vi "Class Method Property File Paths.vi"(8 "error in (no error)":errorcluster) -> (0 "error out":errorcluster, 1 "Method Ini":path, 2 "Property Ini":path, 3 "Class Ini":path, 4 "Files Found Cluster":T1)   [LabVIEW 2023]
doc: "Return paths to class/property/methods xml support files based on the current LV version"
uses:
  <userlib>/_OpenG.lib/file/file.llb/openg_file.lvlib
panel:
  out "file names":string[](array[string])
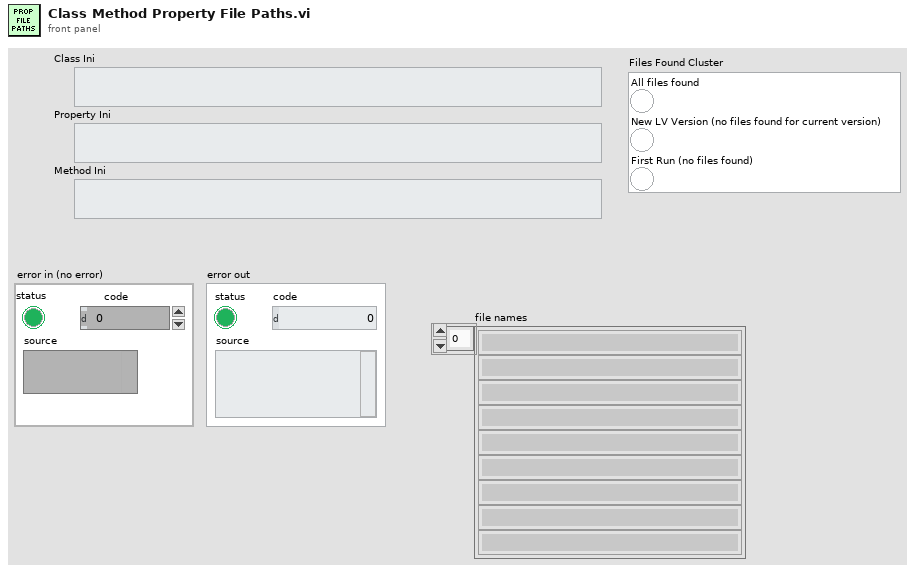
[diagram p1: front panel]
types:
  T1 = cluster{"All files found":bool, "New LV Version (no files found for current version)":bool, "First Run (no files found)":bool}
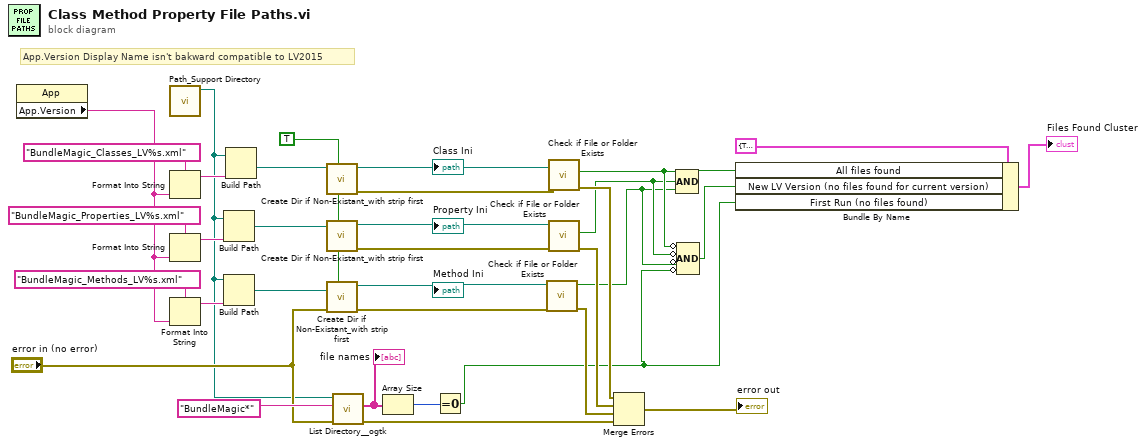
[diagram p0: block diagram]
diagram:
  w25 = TRUE ("Strip Path First [F]")
  # "App.Version Display Name isn't bakward compatible to LV2015"
  n1 = property class="App"() -> ("App.Version"=w35:string)  [unwired: 2 in, 2 out]
  n2 = call "Path_Support Directory.vi"() -> ("Support Directory"=w7:path)  [unwired: 11 in]
  n3 = Format Into String(format string="BundleMagic_Classes_LV%s.xml", w35) -> (resulting string=w30:string)  [unwired: 2 in, 1 out]
  n4 = Format Into String(format string="BundleMagic_Properties_LV%s.xml", w35) -> (resulting string=w31:string)  [unwired: 2 in, 1 out]
  n5 = Format Into String(format string="BundleMagic_Methods_LV%s.xml", w35) -> (resulting string=w34:string)  [unwired: 2 in, 1 out]
  n6 = Build Path(base path=w7, name or relative path=w31) -> (appended path=w27:path)
  n7 = Build Path(base path=w7, name or relative path=w34) -> (appended path=w26:path)
  n8 = Build Path(base path=w7, name or relative path=w30) -> (appended path=w28:path)
  n9 = call "Create Dir if Non-Existant_with strip first.vi"("Strip Path First [F]"=w25, "Directory Path"=w28) -> ("error out"=w21:errorcluster, "dup Directory Path"=w24:path)  [unwired: 7 in, 1 out]
  "Class Ini" <- w24
  n10 = call "Create Dir if Non-Existant_with strip first.vi"("Strip Path First [F]"=w25, "Directory Path"=w27) -> ("error out"=w20:errorcluster, "dup Directory Path"=w23:path)  [unwired: 7 in, 1 out]
  "Property Ini" <- w23
  n11 = call "Create Dir if Non-Existant_with strip first.vi"("Strip Path First [F]"=w25, "error in (no error)"="error in (no error)", "Directory Path"=w26) -> ("error out"=w19:errorcluster, "dup Directory Path"=w22:path)  [unwired: 6 in, 1 out]
  "Method Ini" <- w22
  n12 = call <userlib>:"List Directory__ogtk.vi"("error in (no error)"="error in (no error)", "pattern"="BundleMagic*", "directory path"=w7) -> ("error out"=w9:errorcluster, "file names"=w6:string[])  [unwired: 1 in, 2 out]
  "file names" <- w6
  n13 = Array Size(array=w6) -> (size(s)=w8:i32)
  n14 = Equal To 0?(x=w8) -> (x = 0?=w1:bool)
  n15 = call <vilib>:"Check if File or Folder Exists.vi"("error in (no error)"=w19, "path"=w22) -> ("error out"=w16:errorcluster, "file or folder exists?"=w12:bool)  [unwired: 7 in, 1 out]
  n16 = call <vilib>:"Check if File or Folder Exists.vi"("error in (no error)"=w21, "path"=w24) -> ("error out"=w18:errorcluster, "file or folder exists?"=w14:bool)  [unwired: 7 in, 1 out]
  n17 = call <vilib>:"Check if File or Folder Exists.vi"("error in (no error)"=w20, "path"=w23) -> ("error out"=w17:errorcluster, "file or folder exists?"=w13:bool)  [unwired: 7 in, 1 out]
  n18 = Merge Errors(w18, w17, w16, w9) -> (→"error out":errorcluster)
  n19 = Compound Arithmetic op=AND(w14, w13, w12) -> (w3:bool)
  n20 = Compound Arithmetic op=AND(invert w14, invert w13, invert w12, invert w1) -> (w2:bool)
  n21 = Bundle By Name(cluster=T1 {"All files found"=TRUE, "New LV Version (no files found for current version)"=FALSE, "First Run (no files found)"=FALSE} ("Cluster"), "All files found"=w3, "New LV Version (no files found for current version)"=w2, "First Run (no files found)"=w1) -> (→"Files Found Cluster":T1)
